vi "Numeric LT.vi"(11 "Data In":i32) -> (3 "Data Out":i32)   [LabVIEW 2018]
uses:
  Core/Assert API Components/Failure Actions.ctl
  Core/Assert API Components/Assert API Components.lvlib
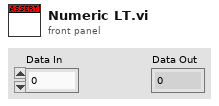
[diagram p1: front panel]
types:
  T1 = typedef "Assert API Components.lvlib/Failure Actions.ctl" = enum16{"None", "Log To File", "Pause Execution", "Abort Execution"}
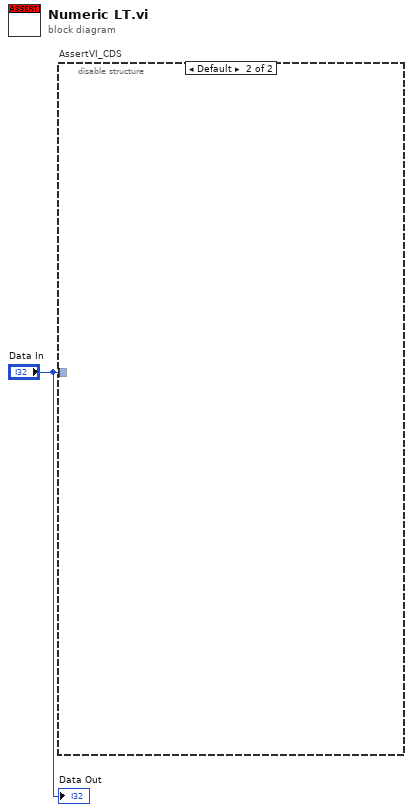
[diagram p0: block diagram]
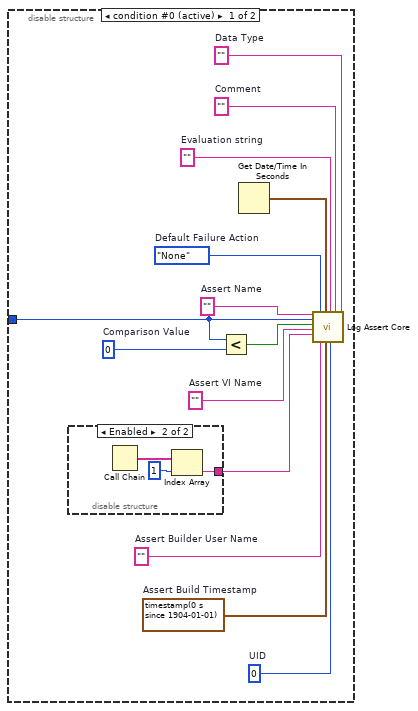
[diagram p2: hidden frame]
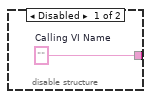
[diagram p3: hidden frame]
diagram:
  n1 = disable-structure "AssertVI_CDS" shown="Default" {
    disable-tunnel: "Data In" -> [w11 _]
    frame condition #0 (active) {
      w3 = 0  # UID
      w5 = ""  # Assert VI Name
      w6 = ""  # Data Type
      w7 = ""  # Assert Builder User Name
      w8 = timestamp(0 s since 1904-01-01)  # Assert Build Timestamp
      w12 = ""  # Comment
      w9 = ""  # Evaluation string
      w14 = Failure_Actions."None"  # Default Failure Action
      w15 = ""  # Assert Name
      w13 = 0  # Comparison Value
      n2 = disable-structure shown="Enabled" {
        disable-tunnel: [w16 w17] -> w2
        frame Disabled {
          w16 = ""  # Calling VI Name
        }
        frame Enabled {
          n3 = Call Chain() -> (call chain=w18:string[])
          n4 = Index Array(array=w18, index=1) -> (element=w17:string)
        }
      }
      n5 = Less?(x=w11, y=w13) -> (x < y?=w10:bool)
      n6 = Get Date/Time In Seconds() -> (seconds since 1Jan1904=w4:timestamp)
      n7 = call "Log Assert Core.vi"("Assert Name"=w15, "Data Value"=w11, "Status"=w10, "Assert VI Name"=w5, "Calling VI Name"=w2, "Failure Action"=w14, "Assert Builder User Name"=w7, "Last Update"=w4, "Assert Build Timestamp"=w8, "Evaluation String"=w9, "Assert VI UID"=w3, "Comment"=w12, "Data Type"=w6) -> ()  [unwired: 7 in]
    }
    frame condition #1 {
    }
  }
  "Data Out" <- "Data In"
